vi "Process rotator axes info.vi"(10 "Incoming axes info":T2[](array[typedef]) {"ActuatorType" items=["Linear", "Rotator", "Goniometer"]}, 11 "Current axes info":T1(array[cluster])) -> (3 "Axes info":T1(array[cluster]))   [LabVIEW 2024]
uses:
  Subsystem modules/Sample rotator/ctl/Axis status.ctl
  Subsystem modules/Sample rotator/SampleRotator.lvlib
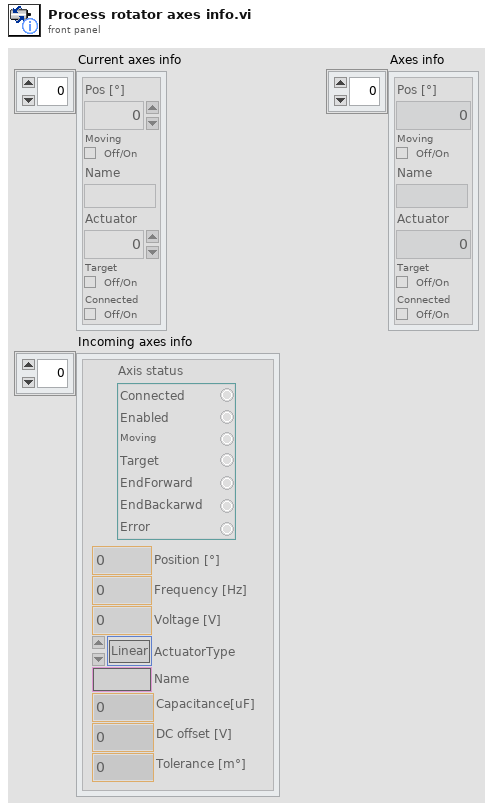
[diagram p1: front panel]
types:
  T1 = cluster{"Pos [°]":dbl, "Moving":bool, "Name":string, "Actuator":u16, "Target":bool, "Connected":bool}[]
  T2 = typedef "SampleRotator.lvlib/Axis status.ctl" = cluster{"Axis status":cluster{"Connected":bool, "Enabled":bool, "Moving":bool, "Target":bool, "EndForward":bool, "EndBackarwd":bool, "Error":bool}, "Position [°]":dbl, "Frequency [Hz]":dbl, "Voltage [V]":dbl, "Capacitance[uF]":dbl, "Name":string, "ActuatorType":u16, "DC offset [V]":dbl, "Tolerance [m°]":dbl}
  T3 = cluster{"Connected":bool, "Enabled":bool, "Moving":bool, "Target":bool, "EndForward":bool, "EndBackarwd":bool, "Error":bool}
  T4 = cluster{"Pos [°]":dbl, "Moving":bool, "Name":string, "Actuator":u16, "Target":bool, "Connected":bool}
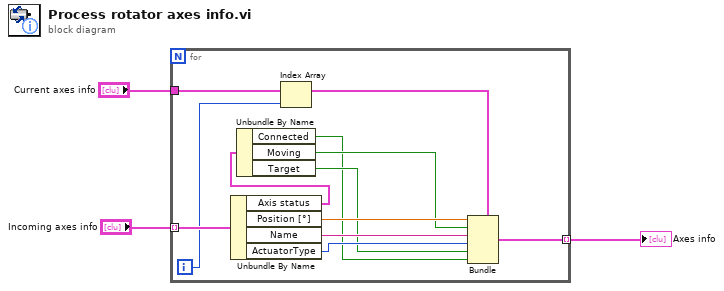
[diagram p0: block diagram]
diagram:
  n1 = for {
    tunnel: "Current axes info" -> [w15]
    tunnel: "Incoming axes info" -> [w12] mode=indexing
    tunnel: [w14] -> w2 mode=indexing
    i -> [w4]
    n2 = Unbundle By Name(w12) -> ("Axis status"=w10:T3, "Position [°]"=w11:dbl, "Name"=w8:string, "ActuatorType"=w7:u16)
    n3 = Unbundle By Name(w10) -> ("Connected"=w5:bool, "Moving"=w9:bool, "Target"=w6:bool)
    n4 = Index Array(array=w15, index=w4) -> (element=w13:T4)
    n5 = Bundle(cluster=w13, "Pos [°]"=w11, "Moving"=w9, "Name"=w8, "Actuator"=w7, "Target"=w6, "Connected"=w5) -> (w14:T4)
  }
  "Axes info" <- w2
